vi "Configure_DMM.vi"(8 "error in (no error)":errorcluster, 10 "DMM_Configuration":T1={"Range"=10.0, "Measurement Type"=enum."DC Volts", "Resolution in Digits"=enum."5 1/2", "pin or relay names"=""} {"Range" format="%.2f"}, 11 "Keysight_34401A-DMM in":refnum<class "Keysight_34401A-DMM.lvclass">) -> (0 "error out":errorcluster, 3 "Keysight_34401A-DMM out":refnum<class "Keysight_34401A-DMM.lvclass">)   [LabVIEW 2020, in "Keysight_34401A-DMM.lvclass"]
uses:
  Keysight_34401A-DMM.lvclass
  DMM_Base/Typedef/DMM_Configuration.ctl
  <instrlib>/Agilent 34401/Agilent 34401.lvlib
  DMM_Base/DMM_Base.lvclass
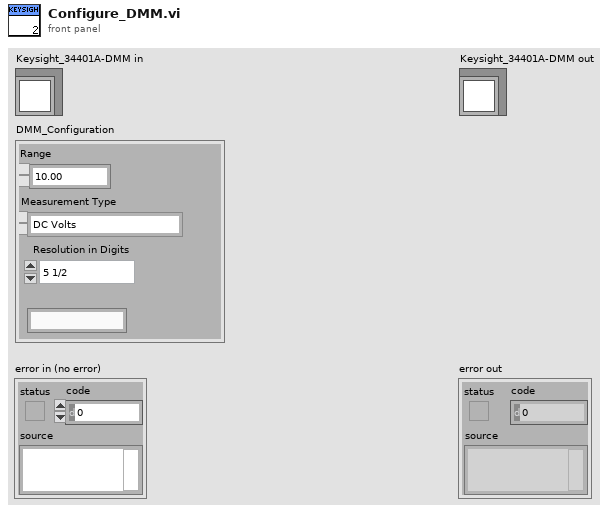
[diagram p1: front panel]
types:
  T1 = typedef "DMM_Base.lvclass/DMM_Configuration.ctl" = cluster{"Range":dbl, "Measurement Type":enum32{"DC Volts", "AC Volts", "DC Current", "AC Current", "2-wire Resistance", "4-wire Resistance", "Diode", "Frequency", "Period", "AC Volts DC Coupled", "Capacitance", "Inductance", "Temperature"}, "Resolution in Digits":enum32{"3 1/2", "4 1/2", "5 1/2", "6 1/2", "7 1/2"}, "pin or relay names":string}
  T2 = enum32{"3 1/2", "4 1/2", "5 1/2", "6 1/2", "7 1/2"}
  T3 = enum32{"DC Volts", "AC Volts", "DC Current", "AC Current", "2-wire Resistance", "4-wire Resistance", "Diode", "Frequency", "Period", "AC Volts DC Coupled", "Capacitance", "Inductance", "Temperature"}
  T4 = typedef "Keysight_34401A-DMM.lvclass/Connection with Session.ctl" = cluster{"connection":T5, "session":refnum<visa-resource-name>}
  T5 = typedef "MeasurementLink Session Management V1.lvlib/Session Reservation.lvclass/Connection.ctl" = cluster{"pin or relay name":string, "site":i32, "instrument type id":string, "channel":string}
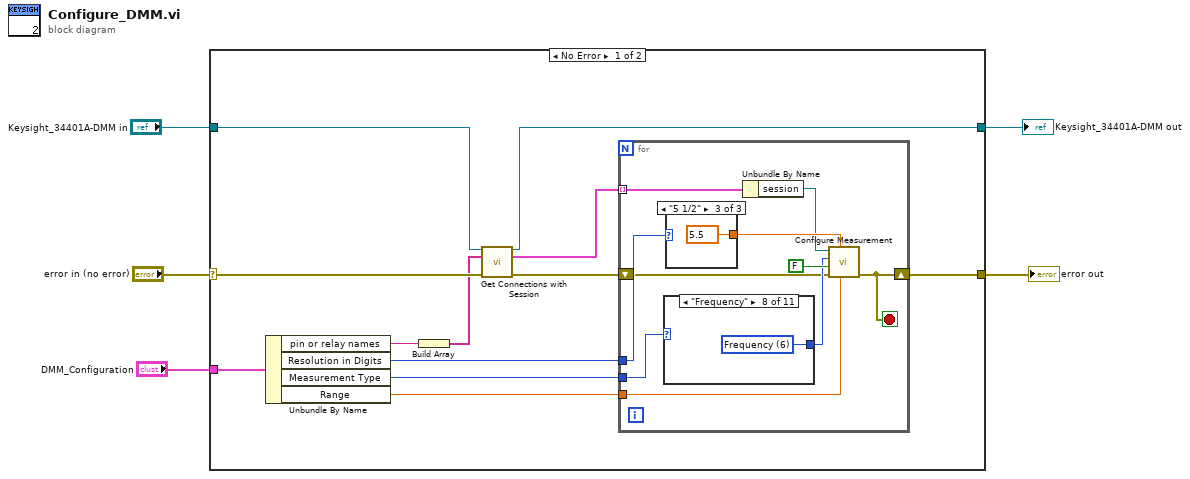
[diagram p0: block diagram]
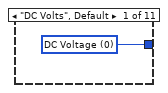
[diagram p2: hidden frame]
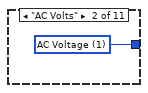
[diagram p3: hidden frame]
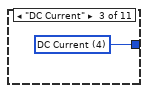
[diagram p4: hidden frame]
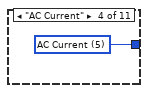
[diagram p5: hidden frame]
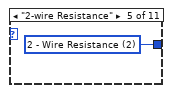
[diagram p6: hidden frame]
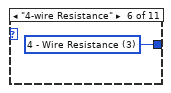
[diagram p7: hidden frame]
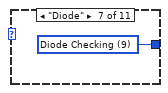
[diagram p8: hidden frame]
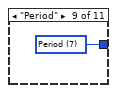
[diagram p9: hidden frame]
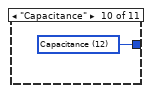
[diagram p10: hidden frame]
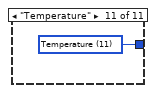
[diagram p11: hidden frame]
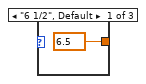
[diagram p12: hidden frame]
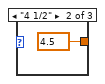
[diagram p13: hidden frame]
diagram:
  n1 = case shown="No Error" "error in (no error)" {
    selector: "error in (no error)" -> [w11 w42]
    tunnel: [w10 w42] -> w4
    tunnel: "Keysight_34401A-DMM in" -> [w9 w43]
    tunnel: [w8 w43] -> w2
    tunnel: "DMM_Configuration" -> [w7 _]
    frame No Error {
      n2 = Unbundle By Name(w7) -> ("pin or relay names"=w14:string, "Resolution in Digits"=w16:T2, "Measurement Type"=w15:T3, "Range"=w17:dbl)
      n3 = Build Array(w14) -> (w6:string[])
      n4 = call "Get Connections with Session.vi"("Keysight_34401A-DMM in"=w9, "pin or relay names"=w6, "error in (no error)"=w11) -> ("Keysight_34401A-DMM out"=w8:refnum<class "Keysight_34401A-DMM.lvclass">, "connections"=w12:T4[], "error out"=w13:errorcluster)  [unwired: 10 in]
      n5 = for {
        tunnel: w17 -> [w27]
        tunnel: w16 -> [w25]
        tunnel: w15 -> [w22]
        shift-right: [w18] -> w10
        shift-left: w13 -> [w21]
        tunnel: w12 -> [w19] mode=indexing
        stop <- w18 stop-if-true
        n6 = case shown="\"Frequency\"" w22 {
          tunnel: [w28 w29 w30 w31 w32 w33 w34 w35 w36 w37 w38] -> w23
          frame "DC Volts", Default {
            w28 = u16 0 items=["DC Voltage", "AC Voltage", "2 - Wire Resistance", "4 - Wire Resistance", "DC Current", "AC Current", "Frequency", "Period", "Continuity", "Diode Checking", "VDC:VDC Ratio", "Temperature", "Capacitance"] ("Function (0: DC Voltage)")
          }
          frame "AC Volts" {
            w29 = u16 1 items=["DC Voltage", "AC Voltage", "2 - Wire Resistance", "4 - Wire Resistance", "DC Current", "AC Current", "Frequency", "Period", "Continuity", "Diode Checking", "VDC:VDC Ratio", "Temperature", "Capacitance"] ("Function (0: DC Voltage)")
          }
          frame "DC Current" {
            w30 = u16 4 items=["DC Voltage", "AC Voltage", "2 - Wire Resistance", "4 - Wire Resistance", "DC Current", "AC Current", "Frequency", "Period", "Continuity", "Diode Checking", "VDC:VDC Ratio", "Temperature", "Capacitance"] ("Function (0: DC Voltage)")
          }
          frame "AC Current" {
            w31 = u16 5 items=["DC Voltage", "AC Voltage", "2 - Wire Resistance", "4 - Wire Resistance", "DC Current", "AC Current", "Frequency", "Period", "Continuity", "Diode Checking", "VDC:VDC Ratio", "Temperature", "Capacitance"] ("Function (0: DC Voltage)")
          }
          frame "2-wire Resistance" {
            w32 = u16 2 items=["DC Voltage", "AC Voltage", "2 - Wire Resistance", "4 - Wire Resistance", "DC Current", "AC Current", "Frequency", "Period", "Continuity", "Diode Checking", "VDC:VDC Ratio", "Temperature", "Capacitance"] ("Function (0: DC Voltage)")
          }
          frame "4-wire Resistance" {
            w33 = u16 3 items=["DC Voltage", "AC Voltage", "2 - Wire Resistance", "4 - Wire Resistance", "DC Current", "AC Current", "Frequency", "Period", "Continuity", "Diode Checking", "VDC:VDC Ratio", "Temperature", "Capacitance"] ("Function (0: DC Voltage)")
          }
          frame "Diode" {
            w34 = u16 9 items=["DC Voltage", "AC Voltage", "2 - Wire Resistance", "4 - Wire Resistance", "DC Current", "AC Current", "Frequency", "Period", "Continuity", "Diode Checking", "VDC:VDC Ratio", "Temperature", "Capacitance"] ("Function (0: DC Voltage)")
          }
          frame "Frequency" {
            w35 = u16 6 items=["DC Voltage", "AC Voltage", "2 - Wire Resistance", "4 - Wire Resistance", "DC Current", "AC Current", "Frequency", "Period", "Continuity", "Diode Checking", "VDC:VDC Ratio", "Temperature", "Capacitance"] ("Function (0: DC Voltage)")
          }
          frame "Period" {
            w36 = u16 7 items=["DC Voltage", "AC Voltage", "2 - Wire Resistance", "4 - Wire Resistance", "DC Current", "AC Current", "Frequency", "Period", "Continuity", "Diode Checking", "VDC:VDC Ratio", "Temperature", "Capacitance"] ("Function (0: DC Voltage)")
          }
          frame "Capacitance" {
            w37 = u16 12 items=["DC Voltage", "AC Voltage", "2 - Wire Resistance", "4 - Wire Resistance", "DC Current", "AC Current", "Frequency", "Period", "Continuity", "Diode Checking", "VDC:VDC Ratio", "Temperature", "Capacitance"] ("Function (0: DC Voltage)")
          }
          frame "Temperature" {
            w38 = u16 11 items=["DC Voltage", "AC Voltage", "2 - Wire Resistance", "4 - Wire Resistance", "DC Current", "AC Current", "Frequency", "Period", "Continuity", "Diode Checking", "VDC:VDC Ratio", "Temperature", "Capacitance"] ("Function (0: DC Voltage)")
          }
        }
        n7 = case shown="\"5 1/2\"" w25 {
          tunnel: [w39 w40 w41] -> w26
          frame "6 1/2", Default {
            w39 = 6.5 items=["4.5"=4.5, "5.5"=5.5, "6.5"=6.5] ("Manual Resolution (5.5 Digits)")
          }
          frame "4 1/2" {
            w40 = 4.5 items=["4.5"=4.5, "5.5"=5.5, "6.5"=6.5] ("Manual Resolution (5.5 Digits)")
          }
          frame "5 1/2" {
            w41 = 5.5 items=["4.5"=4.5, "5.5"=5.5, "6.5"=6.5] ("Manual Resolution (5.5 Digits)")
          }
        }
        n8 = Unbundle By Name(w19) -> ("session"=w20:refnum<visa-resource-name>)
        n9 = call <instrlib>:"Configure Measurement.vi"("Manual Range (1.00)"=w27, "Manual Resolution (5.5 Digits)"=w26, "error in (no error)"=w21, "Enable Auto Range (T: Enable)"=FALSE, "Function (0: DC Voltage)"=w23, "VISA resource name"=w20) -> ("error out"=w18:errorcluster)  [unwired: 4 in, 1 out]
      }
    }
    frame Error {
    }
  }
  "error out" <- w4
  "Keysight_34401A-DMM out" <- w2
